vi "populate_volume_cache.vi"(6 "rebuild job list":bool, 8 "error in (no error)":errorcluster, 10 "cache path":path, 11 "cv_vol path":path) -> (0 "error out":errorcluster, 3 "job paths":path[](array[path]))   [LabVIEW 2024, in "Download_Manager.lvlib"]
uses:
  Download_Manager.lvlib
  CV_RESTful_Library/typedefs/local_volume--cluster.ctl
  CV_Shared_Library/volume.type--enum.ctl
  typedefs/volume_details--cluster.ctl
  <vilib>/addons/_JKI.lib/Serialization/JSON/JKI JSON Serialization.lvlib
  CV_Shared_Library/CV_Shared_Library.lvlib
  CV_RESTful_Library/CV_RESTful_Lib.lvlib
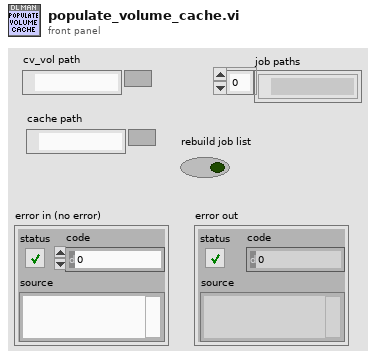
[diagram p1: front panel]
types:
  T1 = typedef "Download_Manager.lvlib/volume_details--cluster.ctl" = cluster{"id":i32, "issue_ids":i32[], "date_last_updated":timestamp}
  T2 = typedef "CV_RESTful_Lib.lvlib/local_volume--cluster.ctl" = cluster{"id":i32, "name":string, "sortable_name":string, "aliases":string[], "description":string, "site_detail_url":string, "count_of_issues":i32, "start_year":i32, "publisher_id":i32, "issue_ids":i32[], "date_last_updated":timestamp, "volume":i32, "cv_id":string, "volume type":T3}
  T3 = typedef "CV_Shared_Library.lvlib/volume.type--enum.ctl" = enum16{"Ongoing", "Limited Series", "Annual", "One Shot", "Reprint/Document", "Star Comics", "Epic Comics"}
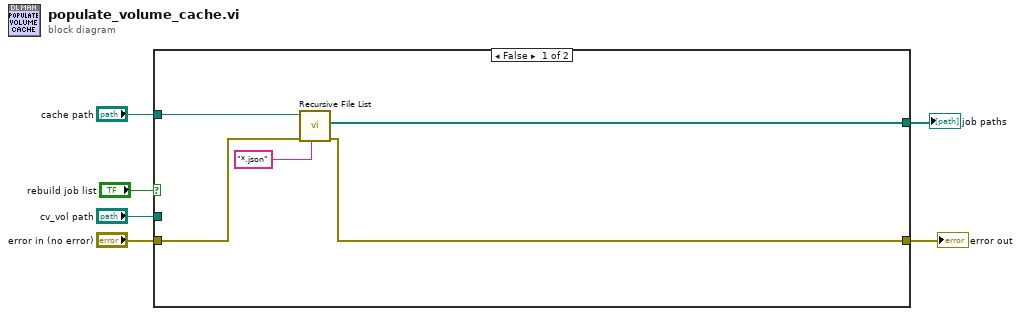
[diagram p0: block diagram]
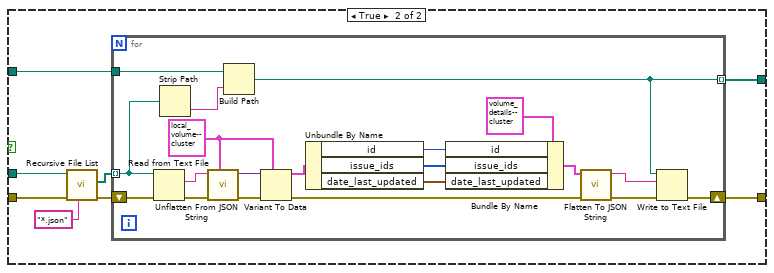
[diagram p2: hidden frame]
diagram:
  n1 = case shown="False" "rebuild job list" {
    tunnel: "cache path" -> [w11 w18]
    tunnel: "cv_vol path" -> [_ w17]
    tunnel: "error in (no error)" -> [w9 w16]
    tunnel: [w8 w13] -> w3
    tunnel: [w7 w12] -> w2
    frame False {
      n2 = call <vilib>:"Recursive File List.vi"("pattern"="*.json", "error in (no error)"=w9, "Folder Path"=w11) -> ("error out"=w8:errorcluster, "All Files in Dir"=w7:path[])  [unwired: 4 in, 3 out]
    }
    frame True {
      n3 = call <vilib>:"Recursive File List.vi"("pattern"="*.json", "error in (no error)"=w16, "Folder Path"=w17) -> ("error out"=w14:errorcluster, "All Files in Dir"=w15:path[])  [unwired: 4 in, 3 out]
      n4 = for {
        tunnel: w15 -> [w37] mode=indexing
        shift-right: [w38] -> w13
        shift-left: w14 -> [w39]
        tunnel: w18 -> [w36]
        tunnel: [w34] -> w12 mode=indexing
        w29 = T2 {"id"=0, "name"="", "sortable_name"="", "aliases"=[], "description"="", "site_detail_url"="", "count_of_issues"=0, "start_year"=0, "publisher_id"=0, "issue_ids"=[], "date_last_updated"=timestamp(0 s since 1904-01-01), "volume"=0, "cv_id"="", "volume type"=enum."One Shot"} ("volume")
        n5 = Read from Text File(file (use dialog)=w37, error in=w39) -> (text=w32:string, error out=w33:errorcluster)  [unwired: 2 in, 2 out]
        n6 = Strip Path(path=w37) -> (name=w35:string)  [unwired: 1 out]
        n7 = call <vilib>:"Unflatten From JSON String.vi"("Type and Defaults"=w29, "error in"=w33, "JSON String"=w32) -> ("error out"=w31:errorcluster, "Variant"=w30:variant)  [unwired: 7 in]
        n8 = Build Path(base path=w36, name or relative path=w35) -> (appended path=w34:path)
        n9 = Variant To Data(error in=w31, type=w29, Variant=w30) -> (data=w28:T2, error out=w23:errorcluster)
        n10 = Unbundle By Name(w28) -> ("id"=w26:i32, "issue_ids"=w25:i32[], "date_last_updated"=w24:timestamp)
        n11 = Bundle By Name(cluster=T1 {"id"=0, "issue_ids"=[], "date_last_updated"=timestamp(0 s since 1904-01-01)} ("volume_details"), "id"=w26, "issue_ids"=w25, "date_last_updated"=w24) -> (w22:T1)
        n12 = call <vilib>:"Flatten To JSON String.vi"("error in"=w23, "Variant"=w22) -> ("error out"=w21:errorcluster, "JSON String"=w20:string)  [unwired: 8 in]
        n13 = Write to Text File(file (use dialog)=w34, text=w20, error in=w21) -> (error out=w38:errorcluster)  [unwired: 1 in, 2 out]
      }
    }
  }
  "error out" <- w3
  "job paths" <- w2
